vi "Aquire Image.vi"(8 "error in (no error)":errorcluster, 9 "Cluster":T1={"Gamma::Value"=1.6, "Gain::Value"=50, "Sharpness::Value"=0, "Contrast::Value"=0.5, "Exposure::Value"=0.0078125} {"Exposure::Value" min=0.000244140625 max=0.5; "Contrast::Value" min=0.0 max=1.0; "Sharpness::Value" min=0 max=2 step=1; "Gain::Value" min=0 max=100 step=1; "Gamma::Value" min=0.01 max=10.0}, 10 "Stop (F)":bool, 11 "QR Code Reader in":refnum<class "QR Code Reader.lvclass">) -> (0 "error out":errorcluster, 2 "Image Out":T2(plugin-control), 3 "QR Code Reader out":refnum<class "QR Code Reader.lvclass">)   [LabVIEW 2021, in "QR Code Reader.lvclass"]
uses:
  QR Code Reader.lvclass
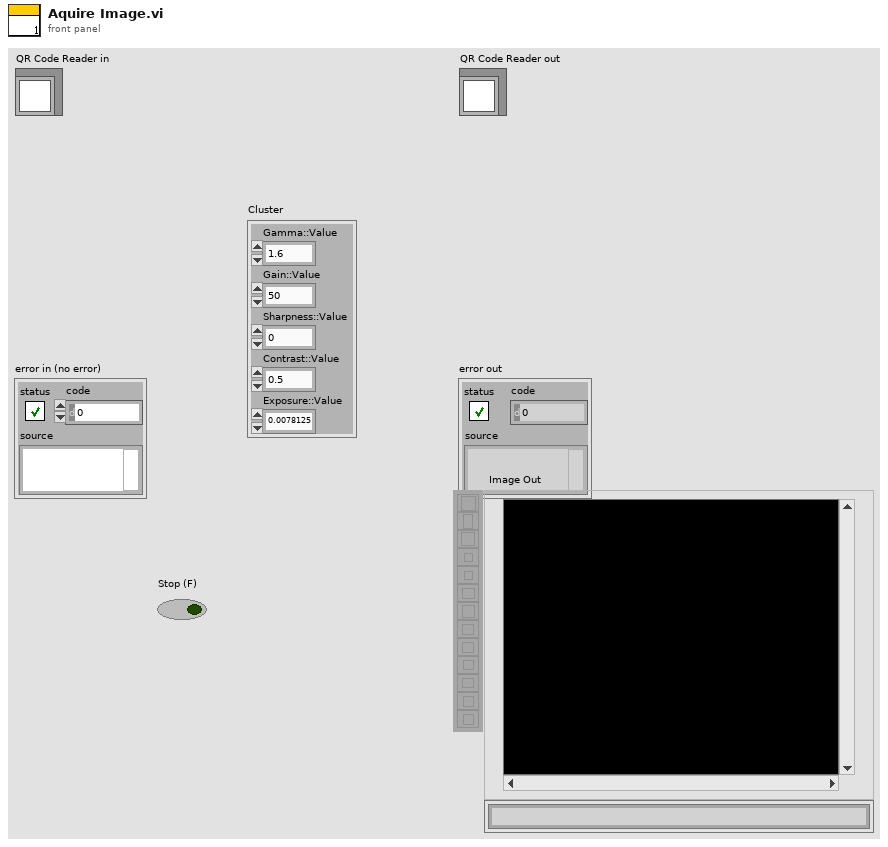
[diagram p1: front panel]
types:
  T1 = cluster{"Gamma::Value":dbl, "Gain::Value":i64, "Sharpness::Value":i64, "Contrast::Value":dbl, "Exposure::Value":dbl}
  T2 = typedef "IMAQ Image.ctl" = refnum<image>
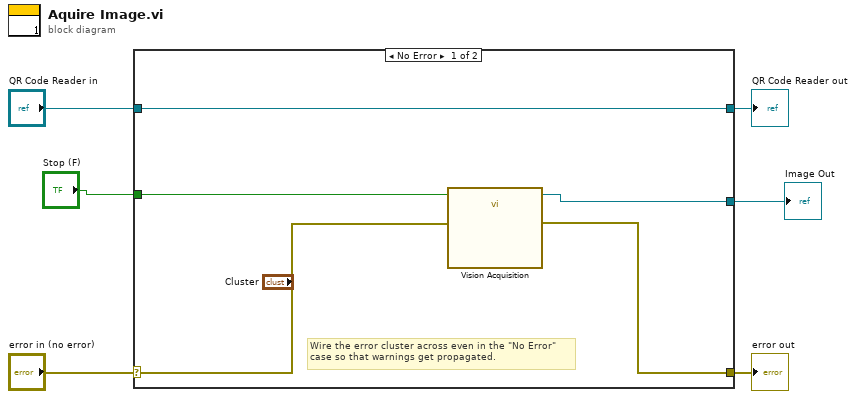
[diagram p0: block diagram]
diagram:
  n1 = case shown="No Error" "error in (no error)" {
    selector: "error in (no error)" -> [w10 w13]
    tunnel: [w9 w13] -> w5
    tunnel: [w11 w12] -> w3
    tunnel: "QR Code Reader in" -> [w11 w12]
    tunnel: [w8 _] -> w2
    tunnel: "Stop (F)" -> [w7 _]
    frame No Error {
      # "Wire the error cluster across even in the \"No Error\"\ncase so that warnings get propagated."
      n2 = call "Vision Acquisition"("Stop (F)"=w7, "error in"=w10) -> ("Image Out"=w8:T2, "error out"=w9:errorcluster)  [unwired: 23 in, 1 out]
    }
    frame Error {
    }
  }
  "error out" <- w5
  "QR Code Reader out" <- w3
  "Image Out" <- w2
